vi "main.vi"() -> ()   [LabVIEW 2012]
uses:
  <vilib>/Utility/file.llb/Write To Spreadsheet File (DBL).vi
panel:
  out "Elapsed Time":dbl format="%#_6f"
  in  "stop":bool
  in  "Output File":path
  out "Latest Point 2":dbl
  out "10 Torr Baratron":dbl[](graph)
  out "Latest Point":dbl
  out "1000 Torr Baratron":dbl[](graph)
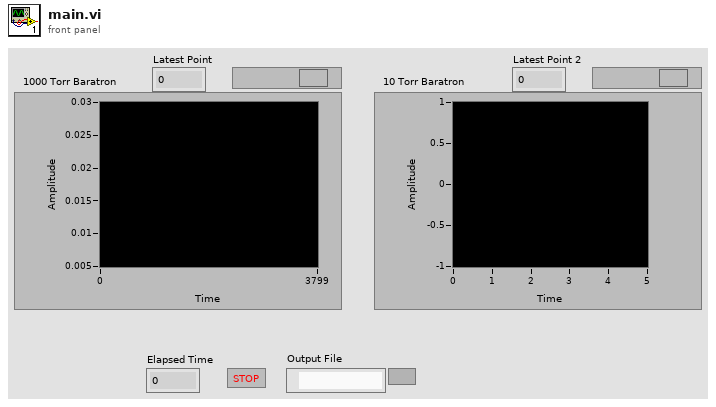
[diagram p1: front panel]
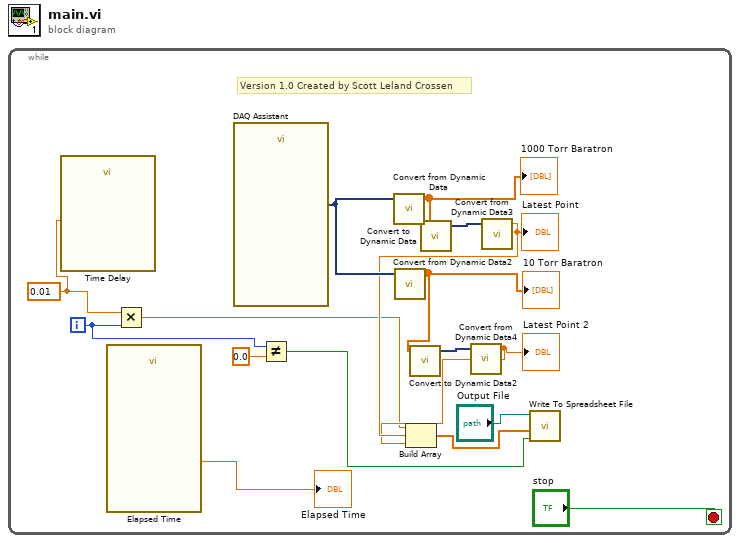
[diagram p0: block diagram]
diagram:
  n1 = while {
    i -> [w2]
    stop <- "stop" stop-if-true
    w4 = 0.01 ("Sample Rate")
    # "Version 1.0 Created by Scott Leland Crossen"
    n2 = call "Time Delay"("Delay Time (s)"=w4) -> ()  [unwired: 10 in, 1 out]
    n3 = call "Elapsed Time"() -> ("Elapsed Time (s)"=→"Elapsed Time":dbl)  [unwired: 12 in, 7 out]
    n4 = Multiply(x=w4, y=w2) -> (x*y=w5:dbl)
    n5 = call "DAQ Assistant"() -> ("data"=w15:dynamicdata)  [unwired: 17 in, 2 out]
    n6 = Not Equal?(x=w2, y=0.0) -> (x != y?=w1:bool)
    n7 = call "Convert from Dynamic Data"("Dynamic Data Type"=w15) -> ("Array"=w14:dbl[])  [unwired: 3 in]
    "1000 Torr Baratron" <- w14
    n8 = call "Convert from Dynamic Data2"("Dynamic Data Type"=w15) -> ("Array"=w11:dbl[])  [unwired: 3 in]
    "10 Torr Baratron" <- w11
    n9 = call "Convert to Dynamic Data2"("Array"=w11) -> ("Dynamic Data Type"=w12:dynamicdata)  [unwired: 3 in]
    n10 = call "Convert to Dynamic Data"("Array"=w14) -> ("Dynamic Data Type"=w13:dynamicdata)  [unwired: 3 in]
    n11 = call "Convert from Dynamic Data4"("Dynamic Data Type"=w12) -> ("Scalar"=w8:dbl)  [unwired: 3 in]
    "Latest Point 2" <- w8
    n12 = call "Convert from Dynamic Data3"("Dynamic Data Type"=w13) -> ("Scalar"=w9:dbl)  [unwired: 3 in]
    "Latest Point" <- w9
    n13 = Build Array(w5, w9, w8) -> (w6:dbl[])
    n14 = call-poly <vilib>:"Write To Spreadsheet File.vi"("append to file? (new file:F)"=w1, "1D data"=w6, "file path (dialog if empty)"="Output File") -> ()  [unwired: 5 in, 1 out]
  }
